vi "SDG60CreateArbWaveformFlatten2.vi"(4 "WFM Source":u16(ring) items=["Single file", "Split files", "Array"], 5 "WFM (Column) Number":i32, 6 "Array WFM":i16[](array[numeric])=[1000, 2000, 3000, 4000, 5000, 6000, 7000, 8000], 7 "WFM Length":i32=15, 8 "error in (no error)":errorcluster, 9 "Timeout (40000 ms)":u32=40000, 10 "Waveform Name (\"wave1\")":string="wave1", 11 "VISA resource name":refnum<visa-resource-name>="USB0::0xF4EC::0x1101::SDG6XEBC5R0119::INSTR") -> (0 "error out":errorcluster, 3 "VISA resource name out":refnum<visa-resource-name>)   [LabVIEW 2018]
doc: "Creates and saves an arbitrary (user-defined) waveform in non-volatile memory, then selects it for output."
uses:
  <vilib>/Utility/file.llb/Read From Spreadsheet File (I64).vi
panel:
  out "Check String":string
  out "WFM to arr time":dbl
  out "Arr to str time":dbl
  out "Upload time":dbl
  out "Total time":dbl
  out "Attempts 0: First":i32
  in  "WFM Path":path=path "C:/Data/_SoftDevelopment/SDG6000/data67107840.txt"
  # "Same vi as with suppliers example,\nbut incorrect negativ case removed.\nInstead calculating twos complement\nexplicitly for negative values.\nThe input range for ARB data is\n-32767..+32767"
  # "Need to set name to be number. not string"
  # "C1 hardcoded as needs to have a channel\nassigned to be uploaded. \nCan then be selected for either channel"
  # "Upon overwrite of name with new WFM, still needs to be selected\notherwise will still use old WFM. If WFM has been selected, and then gets deleted off \nC drive, will still output WFM on that channel"
  # "Max  20E6 (decimal)"
  # "Testing uploads of large WFMS.\n8M: All ok, can have 2 separate WFMs on 2 channels and upload more\n16M: Can have 2 separate WFMs on 2 channels, storage space limits 3rd upload\n          of 16M points, but can upload 8M and switch fine between them all. Can't\n          upload an overwriting 16M point WFM when 2 already saved.\n20M: Can have 20M on both channels, but then no storage space to upload, need to delete\n          old waveform. Upon deletion, can upload 20M and select fine. \n          If two 20M already saved on C, cannot reset and overwrite or just turn off outputs,\n          requires deletion of old waveform\n\nTo overwrite a 20M point WFM, overwrite it with a small WFM, then overwrite with 20M \n\nIf too large a waveform is uploaded, generator will crash requiring manual power cycle"
  # "If storage full, will beep on machine-say storage full, but not give any error through \nlabview. Waveform won't ovewrite others when uploading"
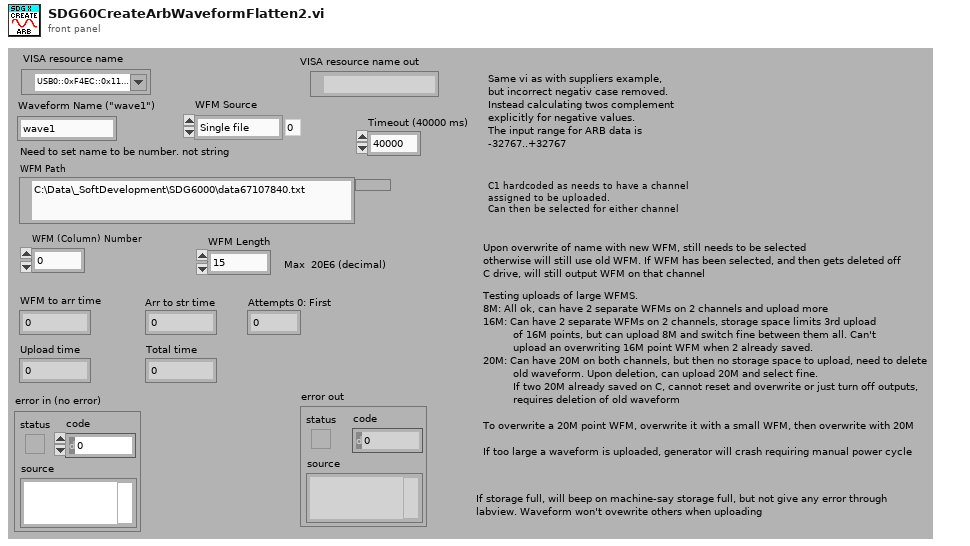
[diagram p1: front panel]
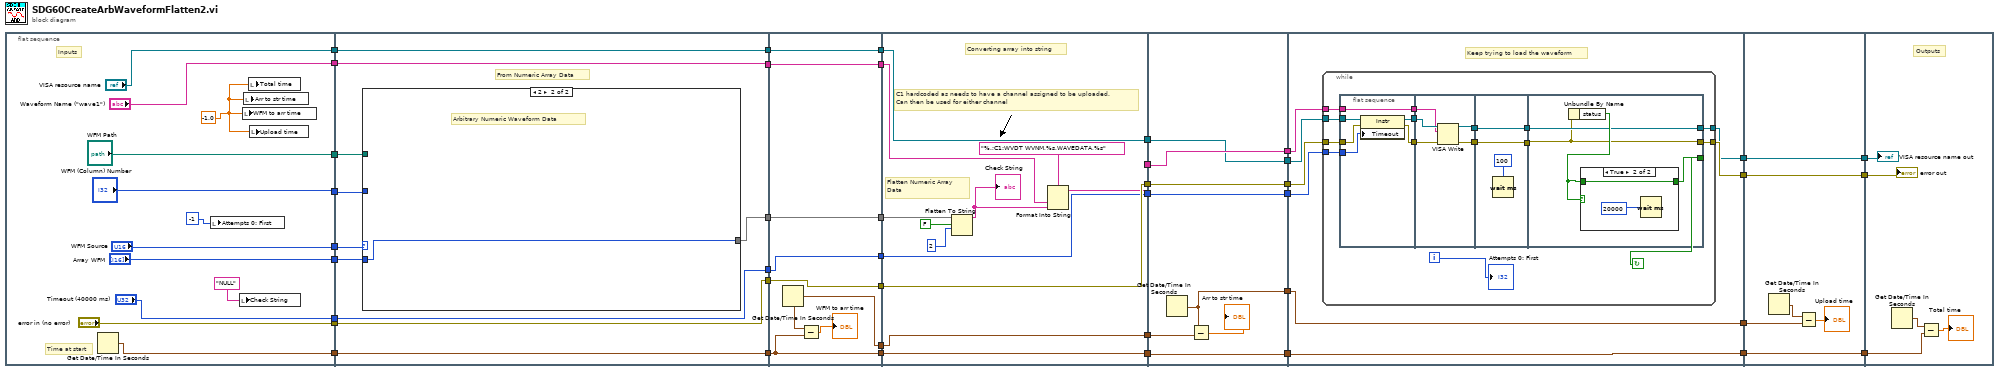
[diagram p0: block diagram]
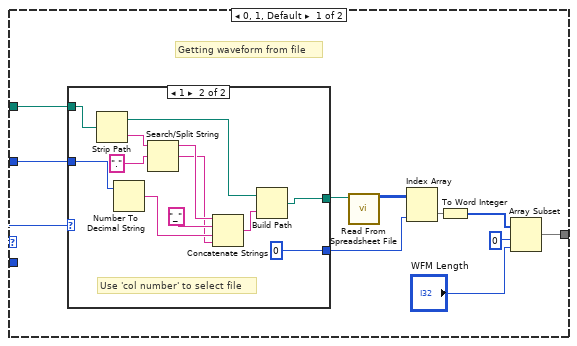
[diagram p2: hidden frame]
diagram:
  n1 = flat-sequence {
    tunnel: ["WFM Source"] -> w41
    tunnel: ["Array WFM"] -> w40
    tunnel: ["WFM Path"] -> w39
    tunnel: ["WFM (Column) Number"] -> w38
    tunnel: ["VISA resource name"] -> w37
    tunnel: ["Waveform Name (\"wave1\")"] -> w36
    tunnel: ["error in (no error)"] -> w35
    tunnel: ["Timeout (40000 ms)"] -> w34
    tunnel: [w45] -> w33
    tunnel: w41 -> [w63]
    tunnel: w40 -> [w62]
    tunnel: [w61] -> w32
    tunnel: w39 -> [w60]
    tunnel: w38 -> [w59]
    tunnel: [w58] -> w30
    tunnel: w37 -> [w58]
    tunnel: [w57] -> w28
    tunnel: w36 -> [w57]
    tunnel: [w56] -> w26
    tunnel: w35 -> [w56]
    tunnel: [w55] -> w24
    tunnel: w34 -> [w55]
    tunnel: [w54] -> w22
    tunnel: w33 -> [w54]
    tunnel: w32 -> [w97]
    tunnel: [w97] -> w31
    tunnel: w30 -> [w96]
    tunnel: [w96] -> w29
    tunnel: w28 -> [w95]
    tunnel: [w95] -> w27
    tunnel: w26 -> [w91]
    tunnel: [w91] -> w25
    tunnel: w24 -> [w92]
    tunnel: [w92] -> w23
    tunnel: w22 -> [w93]
    tunnel: [w93] -> w21
    tunnel: [w90] -> w1
    tunnel: w31 -> [w100]
    tunnel: [w102] -> w20
    tunnel: [w108] -> w18
    tunnel: [w107] -> w16
    tunnel: [w106] -> w14
    tunnel: w29 -> [w108]
    tunnel: w27 -> [w105]
    tunnel: w25 -> [w107]
    tunnel: w23 -> [w106]
    tunnel: w21 -> [w104]
    tunnel: [w104] -> w12
    tunnel: [w103] -> w2
    tunnel: w1 -> [w103]
    tunnel: w20 -> [w117]
    tunnel: [w117] -> w19
    tunnel: w18 -> [w116]
    tunnel: [w116] -> w17
    tunnel: w16 -> [w115]
    tunnel: [w115] -> w15
    tunnel: w14 -> [w114]
    tunnel: [w114] -> w13
    tunnel: w12 -> [w110]
    tunnel: [w110] -> w11
    tunnel: [w112] -> w4
    tunnel: w2 -> [w111]
    tunnel: [w121] -> w10
    tunnel: [w120] -> w8
    tunnel: w19 -> [w125]
    tunnel: w17 -> [w124]
    tunnel: w15 -> [w123]
    tunnel: w13 -> [w122]
    tunnel: w11 -> [w119]
    tunnel: [w119] -> w6
    tunnel: w4 -> [w118]
    tunnel: [w118] -> w3
    tunnel: w10 -> [w167]
    tunnel: [w167] -> w9
    tunnel: w8 -> [w166]
    tunnel: [w166] -> w7
    tunnel: w6 -> [w164]
    tunnel: [w164] -> w5
    tunnel: w3 -> [w163]
    tunnel: w9 -> [w172]
    tunnel: w7 -> [w171]
    tunnel: w5 -> [w168]
    frame #0 {
      w44 = -1.0
      # "Inputs"
      # "Time at start"
      n2 = Get Date/Time In Seconds() -> (seconds since 1Jan1904=w45:timestamp)
      n3 = local write "Attempts 0: First"(-1) -> ()
      n4 = local write "Check String"("NULL") -> ()
      n5 = local write "WFM to arr time"(w44) -> ()
      n6 = local write "Arr to str time"(w44) -> ()
      n7 = local write "Total time"(w44) -> ()
      n8 = local write "Upload time"(w44) -> ()
    }
    frame #1 {
      # "From Numeric Array Data"
      n9 = case shown="2" w63 {
        selector: w63 -> [w72 _]
        tunnel: [w67 w89] -> w61
        tunnel: w62 -> [_ w89]
        tunnel: w60 -> [w66 _]
        tunnel: w59 -> [w65 _]
        frame 0, 1, Default {
          # "Getting waveform from file"
          n10 = case shown="1" w72 {
            tunnel: w66 -> [w76 w88]
            tunnel: w65 -> [w75 w85]
            tunnel: [w76 w78] -> w70
            tunnel: [w75 0 ("x")] -> w69
            frame 0, Default {
              # "File contains multiple wfms"
            }
            frame 1 {
              # "Use 'col number' to select file"
              n11 = Strip Path(path=w88) -> (stripped path=w80:path, name=w86:string)
              n12 = Number To Decimal String(number=w85) -> (decimal integer string=w82:string)  [unwired: 1 in]
              n13 = Search/Split String(string=w86, search string/char (-)=".") -> (substring before match=w84:string, match + rest of string=w81:string)  [unwired: 1 in, 1 out]
              n14 = Concatenate Strings(w84, "_", w82, w81) -> (w79:string)
              n15 = Build Path(base path=w80, name or relative path=w79) -> (appended path=w78:path)
            }
          }
          n16 = call-poly <vilib>:"Read From Spreadsheet File.vi"("file path (dialog if empty)"=w70) -> ("all rows"=w71:i64[][])  [unwired: 6 in, 4 out]
          n17 = Index Array(array=w71, index (col)=w69) -> (element=w68:i64[])  [unwired: 1 in]
          n18 = To Word Integer(number=w68) -> (16bit integer=w74:i16[])
          n19 = Array Subset(array=w74, index=0 ("x"), length="WFM Length") -> (w67:i16[])
        }
        frame 2 {
          # "Arbitrary Numeric Waveform Data"
        }
      }
    }
    frame #2 {
      n20 = Get Date/Time In Seconds() -> (seconds since 1Jan1904=w90:timestamp)
      n21 = Subtract(x=w90, y=w93) -> (x-y=→"WFM to arr time":dbl)
    }
    frame #3 {
      # "Converting array into string"
      # "C1 hardcoded as needs to have a channel assigned to be uploaded. \nCan then be used for either channel"
      # "Flatten Numeric Array \nData"
      n22 = Flatten To String(anything=w100, prepend array or string size? (T)=FALSE, byte order (0:big-endian, network order)=2) -> (data string=w98:string)  [unwired: 1 in, 2 out]
      "Check String" <- w98
      n23 = Format Into String(format string="%.;C1:WVDT WVNM,%s,WAVEDATA,%s", w105, w98) -> (resulting string=w102:string)  [unwired: 2 in, 1 out]
    }
    frame #4 {
      n24 = Get Date/Time In Seconds() -> (seconds since 1Jan1904=w112:timestamp)
      n25 = Subtract(x=w112, y=w111) -> (x-y=→"Arr to str time":dbl)
    }
    frame #5 {
      # "Keep trying to load the waveform"
      n26 = while {
        tunnel: w125 -> [w140]
        tunnel: w124 -> [w139]
        tunnel: w123 -> [w138]
        tunnel: [w137] -> w121
        tunnel: [w136] -> w120
        tunnel: w122 -> [w126]
        i -> [w132]
        stop <- w135 continue-if-true
        n27 = flat-sequence {
          tunnel: w140 -> [w146]
          tunnel: w138 -> [w143]
          tunnel: w139 -> [w145]
          tunnel: [w144] -> w129
          tunnel: [w142] -> w128
          tunnel: [w146] -> w127
          tunnel: w126 -> [w141]
          tunnel: [w147] -> w134
          tunnel: [w148] -> w133
          tunnel: w129 -> [w150]
          tunnel: w128 -> [w151]
          tunnel: w127 -> [w149]
          tunnel: w134 -> [w152]
          tunnel: w133 -> [w153]
          tunnel: [w153] -> w131
          tunnel: [w152] -> w130
          tunnel: [w156] -> w136
          tunnel: [w155] -> w137
          tunnel: [w157] -> w135
          tunnel: w131 -> [w156]
          tunnel: w130 -> [w155]
          frame #0 {
            n28 = property class="Instr"(reference=w145, error in=w143, "Timeout"=w141) -> (reference out=w144:refnum<visa-resource-name>, error out=w142:errorcluster)
          }
          frame #1 {
            n29 = VISA Write(VISA resource name=w150, write buffer=w149, error in (no error)=w151) -> (VISA resource name out=w148:refnum<visa-resource-name>, error out=w147:errorcluster)  [unwired: 1 out]
          }
          frame #2 {
            n30 = Wait (ms)(milliseconds to wait=100 ("x")) -> ()  [unwired: 1 out]
          }
          frame #3 {
            n31 = Unbundle By Name(w155) -> ("status"=w158:bool)
            n32 = case shown="True" w158 {
              tunnel: w158 -> [w159 w160]
              tunnel: [w159 w160] -> w157
              frame False {
              }
              frame True {
                n33 = Wait (ms)(milliseconds to wait=20000 ("x")) -> ()  [unwired: 1 out]
              }
            }
          }
        }
        "Attempts 0: First" <- w132
      }
    }
    frame #6 {
      n34 = Get Date/Time In Seconds() -> (seconds since 1Jan1904=w165:timestamp)
      n35 = Subtract(x=w165, y=w163) -> (x-y=→"Upload time":dbl)
    }
    frame #7 {
      # "Outputs"
      n36 = Get Date/Time In Seconds() -> (seconds since 1Jan1904=w170:timestamp)
      n37 = Subtract(x=w170, y=w168) -> (x-y=→"Total time":dbl)
      "VISA resource name out" <- w171
      "error out" <- w172
    }
  }
